vi "cloud_connection_arduino_uno.vi"() -> ()   [LabVIEW 2020]
uses:
  <vilib>/Skyline/Tag/Shared/typedefs/DataType.ctl
  <vilib>/Skyline/Tag/Wrapper/Wrapper_class/Tag Value Cluster Wrapper.ctl
  <vilib>/Skyline/Configuration/Configuration_class/NI Skyline Configuration.lvclass
  <vilib>/Skyline/Tag/Shared/typedefs/Tag Value Cluster.ctl
  <vilib>/Skyline/Tag/Wrapper/Wrapper_class/Generate Tag Cluster (DBL) 2.vi
  <vilib>/Skyline/Tag/Shared/Serialize Double to String.vi
  <vilib>/MakerHub/LINX/Public/Utilities/Open Serial.vi
  <vilib>/MakerHub/LINX/Public/Sensors/Motion/Servo/Servo Open One Channel.vi
  <vilib>/Skyline/Configuration/Configuration HTTP_class/Open Configuration API Key.vi
  <vilib>/Skyline/Tag/Wrapper/Wrapper_class/Configure Retention (Count).vi
  <vilib>/MakerHub/LINX/Public/Sensors/Motion/Servo/Servo Set Pulse Width One Channel.vi
  <vilib>/Utility/file.llb/Read Delimited Spreadsheet (DBL).vi
  <vilib>/Skyline/Tag/Wrapper/Wrapper_class/Generate Tag Cluster Core 2.vi
  <vilib>/MakerHub/LINX/Public/Sensors/Motion/Servo/Servo Close One Channel.vi
  <vilib>/Skyline/Tag/Wrapper/Wrapper_class/Close Tag (Multiple).vi
  <vilib>/Skyline/Configuration/Configuration HTTP_class/NI Skyline Configuration HTTP.lvclass
  <vilib>/Skyline/Tag/Wrapper/Wrapper HTTP_class/NI Skyline Tag HTTP.lvclass
  <vilib>/Skyline/Tag/Wrapper/Wrapper_class/NI Skyline Tag.lvclass
  <vilib>/Skyline/Tag/Shared/NI Skyline Tag.lvlib
  <vilib>/MakerHub/LINX/LMH-LINX.lvlib
  <vilib>/MakerHub/LINX/Public/Sensors/Motion/Servo/Servo.lvlib
panel:
  out "Angle1":dbl format="%#_3f"
  out "Angle2":dbl
  out "Angle 3":dbl
  in  "start 2":bool
  out "Error Out 2":errorcluster
  out "Error Out":errorcluster
  in  "Serial Port":refnum<visa-resource-name>="N/A"
  out "size(s)":i32
  out "subarray":dbl[](array[numeric])
  out "all rows":dbl[][](array[numeric])
  in  "start":bool
  in  "stop":bool
  in  "error in (no error)":errorcluster
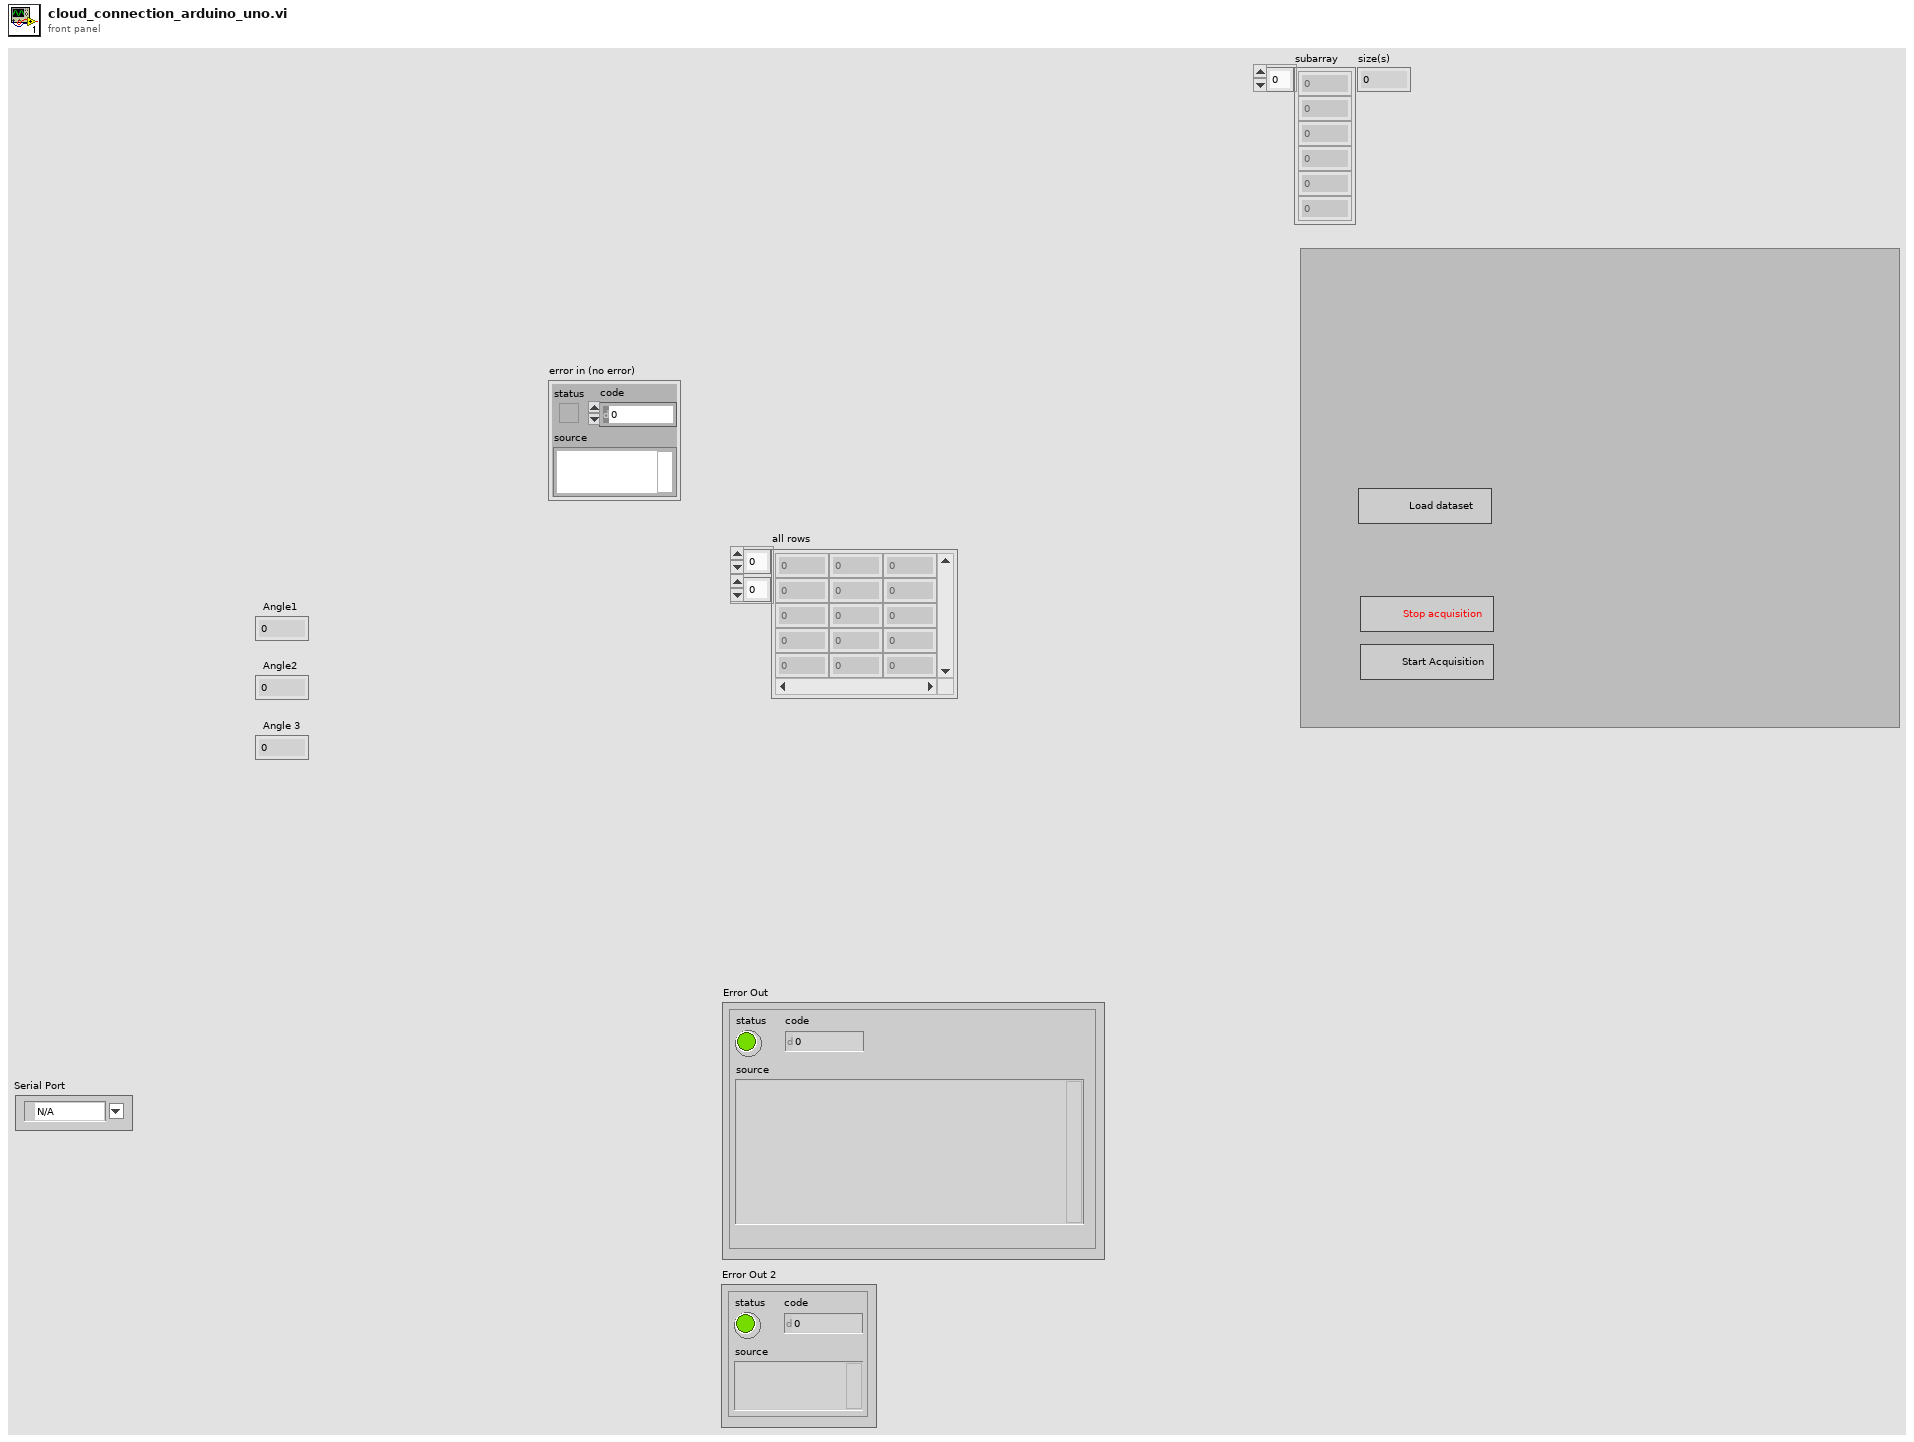
[diagram p1: front panel]
types:
  T1 = typedef "NI Skyline Tag.lvlib/DataType.ctl" = enum32{"Double", "I32", "String", "Boolean", "U64", "Timestamp"}
  T2 = typedef "LMH-LINX.lvlib/LINX Ref.ctl" = cluster{"IO":T3, "Interface":T4, "LINX Device Config":T5}
  T3 = typedef "LMH-LINX.lvlib/Platform.ctl" = enum16{"Remote", "Local"}
  T4 = typedef "LMH-LINX.lvlib/Interface.ctl" = enum16{"Serial", "TCP"}
  T5 = typedef "LMH-LINX.lvlib/Device.lvlib/LINX Device Config.ctl" = cluster{"Interface":T4, "COM Port":refnum<visa-resource-name>, "TCP Configuration":T6, "Device Family":u8, "Device ID":u8, "Device Name":string, "TCP Ref":refnum<k5>, "Channels":T7}
  T6 = typedef "LMH-LINX.lvlib/Device.lvlib/TCP Config.ctl" = cluster{"IP Address":string, "Port":u16}
  T7 = typedef "LMH-LINX.lvlib/Channels.ctl" = cluster{"DI":u8[], "DO":u8[], "AI":u8[], "AO":u8[], "PWM":u8[], "QE":u8[], "UART":u8[], "I2C 2":u8[], "SPI":u8[], "CAN":u8[], "Servo":u8[], "AI Ref (V)":dbl, "AI Resolution (Bits)":u8, "AO Ref (V)":dbl, "AO Resolution (Bits)":u8}
  T8 = typedef "NI Skyline Tag.lvclass/Tag Value Cluster Wrapper.ctl" = cluster{"Configuration":refnum<class "NI Skyline Configuration.lvclass">, "Tag Cluster":T9}
  T9 = typedef "NI Skyline Tag.lvlib/Tag Value Cluster.ctl" = cluster{"Path":string, "Workspace ID":string, "Data Type":T1, "Value":string, "Time Stamp":timestamp}
  T10 = cluster{"[0]":dbl, "[1]":dbl, "[2]":dbl, "[3]":dbl, "[4]":dbl, "[5]":dbl, "[6]":dbl, "[7]":dbl, "[8]":dbl}
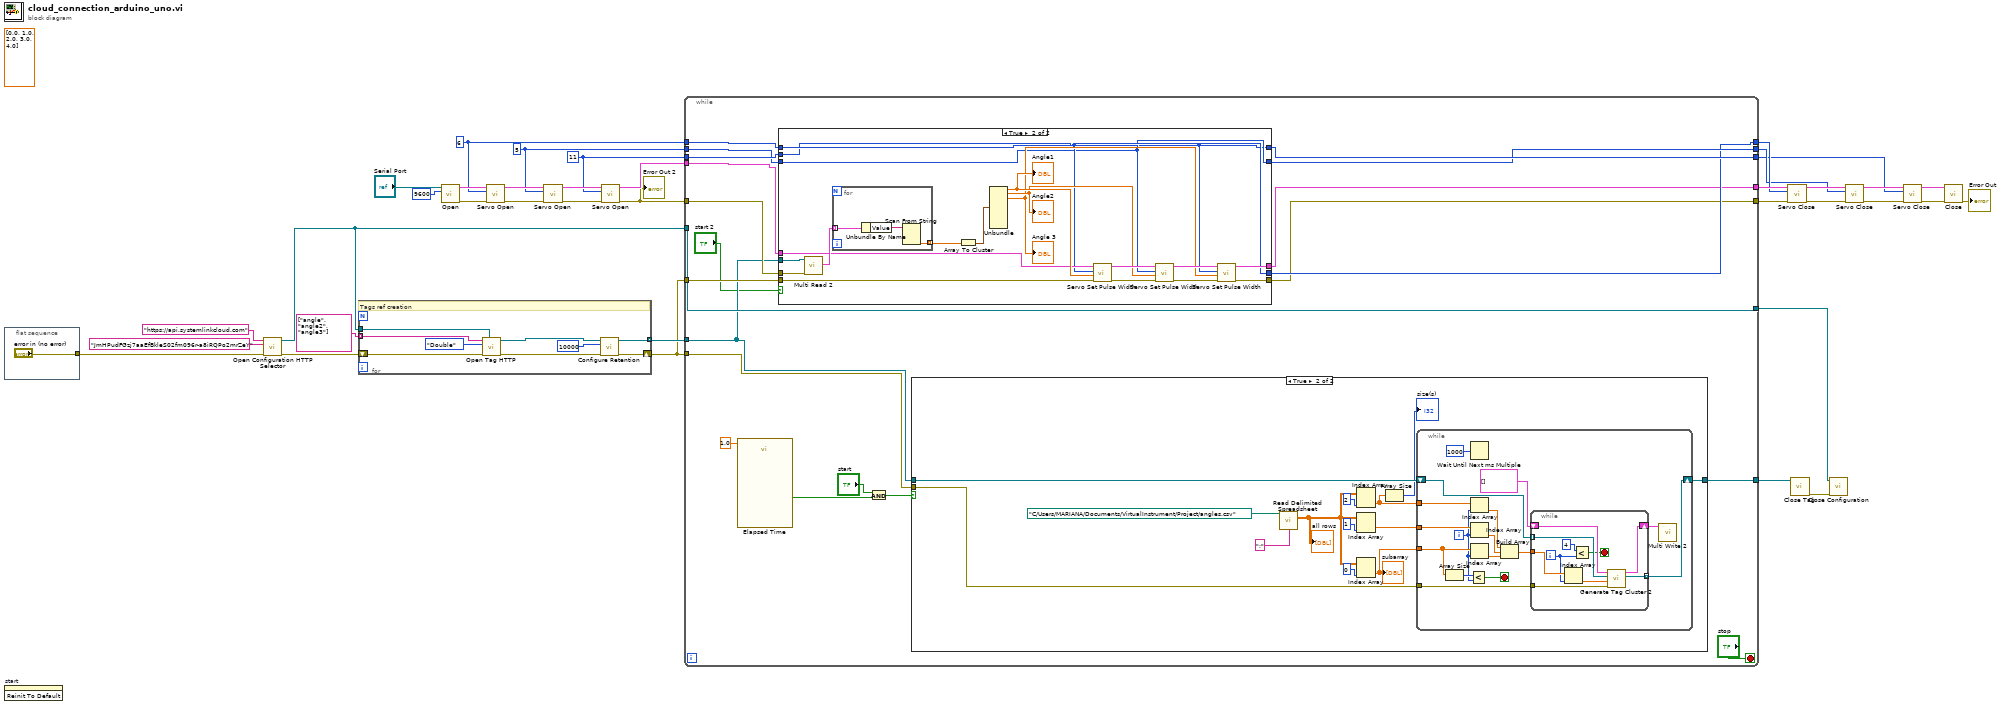
[diagram p0: block diagram]
diagram:
  w3 = u8 11 ("Servo Channel")
  w5 = u8 5 ("Servo Channel")
  w7 = u8 6 ("Servo Channel")
  (unwired) dbl[] [0.0, 1.0, 2.0, 3.0, 4.0]
  n1 = flat-sequence {
    tunnel: ["error in (no error)"] -> w34
    frame #0 {
    }
  }
  n2 = invoke on="start" class="Bool (strict)" method="Reinit To Default"() -> ()  [unwired: 3 in, 3 out]
  n3 = call-poly <vilib>:"Open Configuration HTTP Selector.vi"("error in (no error)"=w34, "api key"="JmHPudFGzj7aaEfBkleS02fm096r-a8iRQPo2mrZeY", "server url"="https://api.systemlinkcloud.com") -> ("error out"=w33:errorcluster, "configuration"=w30:refnum<class "NI Skyline Configuration HTTP.lvclass">)  [unwired: 7 in]
  n4 = for "Tags ref or creation" {
    tunnel: w30 -> [w46]
    tunnel: [w43] -> w29 mode=indexing
    tunnel: string[] ["angle", "angle2", "angle3"] -> [w38] mode=indexing
    shift-right: [w39] -> w1
    shift-left: w33 -> [w42]
    # "Tags ref creation"
    n5 = call <vilib>:"Open Tag HTTP.vi"("configuration"=w46, "error in (no error)"=w42, "Data Type"=DataType."Double", "path"=w38) -> ("error out"=w40:errorcluster, "tag"=w45:refnum<class "NI Skyline Tag.lvclass">)  [unwired: 6 in]
    n6 = call-poly <vilib>:"Configure Retention.vi"("error in (no error)"=w40, "maximum count"=u32 10000, "tag in"=w45) -> ("error out"=w39:errorcluster, "tag out"=w43:refnum<class "NI Skyline Tag.lvclass">)  [unwired: 7 in]
  }
  n7 = call-poly <vilib>:"Open.vi"("Baud Rate Override"=u32 9600, "Serial Port"="Serial Port") -> ("Error Out"=w25:errorcluster, "LINX Resource"=w26:T2)  [unwired: 7 in, 1 out]
  n8 = call-poly <vilib>:"Servo Open.vi"("Error In"=w25, "Servo Channel"=w7, "LINX Resource"=w26) -> ("Error Out"=w21:errorcluster, "LINX Resource"=w22:T2)  [unwired: 7 in]
  n9 = call-poly <vilib>:"Servo Open.vi"("Error In"=w21, "Servo Channel"=w5, "LINX Resource"=w22) -> ("Error Out"=w16:errorcluster, "LINX Resource"=w17:T2)  [unwired: 7 in]
  n10 = call-poly <vilib>:"Servo Open.vi"("Error In"=w16, "Servo Channel"=w3, "LINX Resource"=w17) -> ("Error Out"=w8:errorcluster, "LINX Resource"=w9:T2)  [unwired: 7 in]
  "Error Out 2" <- w8
  n11 = while {
    tunnel: [w67] -> w31
    tunnel: w30 -> [w67]
    tunnel: w1 -> [w60]
    tunnel: w29 -> [w53]
    tunnel: [w66] -> w27
    tunnel: [w49] -> w11
    tunnel: [w48] -> w10
    tunnel: w9 -> [w56]
    tunnel: w8 -> [w55]
    tunnel: w7 -> [w57]
    tunnel: [w50] -> w6
    tunnel: w5 -> [w58]
    tunnel: [w51] -> w4
    tunnel: w3 -> [w59]
    tunnel: [w52] -> w2
    tunnel: w1 -> [w54]
    stop <- "stop" stop-if-true
    n12 = call "Elapsed Time"("Time Target (s)"=1.0) -> ("Time has Elapsed"=w62:bool)  [unwired: 11 in, 7 out]
    n13 = case shown="True" "start 2" {
      tunnel: w53 -> [_ w89]
      tunnel: w55 -> [_ w87]
      tunnel: w59 -> [w70 w73]
      tunnel: w58 -> [w69 w74]
      tunnel: w57 -> [w68 w75]
      tunnel: w56 -> [w72 w79]
      tunnel: w54 -> [w71 w78]
      tunnel: [w72 w77] -> w49
      tunnel: [w71 w76] -> w48
      tunnel: [w70 w75] -> w50
      tunnel: [w69 w74] -> w51
      tunnel: [w68 w73] -> w52
      frame False {
      }
      frame True {
        n14 = call <vilib>:"Multi Read 2.vi"("error in (no error)"=w87, "tags in"=w89) -> ("tag clusters"=w88:T9[])  [unwired: 7 in, 2 out]
        n15 = for {
          tunnel: [w94] -> w91 mode=indexing
          tunnel: w88 -> [w92] mode=indexing
          n16 = Unbundle By Name(w92) -> ("Value"=w93:string)
          n17 = Scan From String(input string=w93) -> (output 1=w94:dbl)  [unwired: 4 in, 3 out]
        }
        n18 = Array To Cluster(array=w91) -> (cluster=w90:T10)
        n19 = Unbundle(w90) -> ("[0]"=w82:dbl, "[1]"=w81:dbl, "[2]"=w80:dbl)  [unwired: 6 out]
        "Angle1" <- w82
        "Angle2" <- w81
        "Angle 3" <- w80
        n20 = call-poly <vilib>:"Servo Set Pulse Width.vi"("Error In"=w78, "Pulse Width (uS)"=w82, "Servo Channel"=w75, "LINX Resource"=w79) -> ("Error Out"=w85:errorcluster, "LINX Resource"=w86:T2)  [unwired: 6 in]
        n21 = call-poly <vilib>:"Servo Set Pulse Width.vi"("Error In"=w85, "Pulse Width (uS)"=w81, "Servo Channel"=w74, "LINX Resource"=w86) -> ("Error Out"=w83:errorcluster, "LINX Resource"=w84:T2)  [unwired: 6 in]
        n22 = call-poly <vilib>:"Servo Set Pulse Width.vi"("Error In"=w83, "Pulse Width (uS)"=w80, "Servo Channel"=w73, "LINX Resource"=w84) -> ("Error Out"=w76:errorcluster, "LINX Resource"=w77:T2)  [unwired: 6 in]
      }
    }
    n23 = And(x="start", y=w62) -> (x .and. y?=w61:bool)
    n24 = case shown="True" w61 {
      tunnel: w60 -> [_ w107]
      tunnel: w53 -> [w95 w106]
      tunnel: [w95 w108] -> w66
      frame False {
      }
      frame True {
        n25 = call-poly <vilib>:"Read Delimited Spreadsheet.vi"("file path (dialog if empty)"=path "C:/Users/MARIANA/Documents/VirtualInstrument/Project/angles.csv", "delimiter (\\t)"=";" ("delimiter (\\t)")) -> ("all rows"=w101:dbl[][])  [unwired: 8 in, 5 out]
        "all rows" <- w101
        n26 = Index Array(array=w101, index (col)=2 ("index")) -> (element=w97:dbl[])  [unwired: 1 in]
        n27 = Index Array(array=w101, index (col)=1 ("index")) -> (element=w100:dbl[])  [unwired: 1 in]
        n28 = Index Array(array=w101, index (col)=0 ("disabled index (col)")) -> (element=w102:dbl[])  [unwired: 1 in]
        "subarray" <- w102
        n29 = Array Size(array=w97) -> (size(s)=→"size(s)":i32)
        n30 = while {
          tunnel: w107 -> [w122]
          shift-right: [w123] -> w108
          shift-left: w106 -> [w120]
          tunnel: w102 -> [w116]
          tunnel: w100 -> [w112]
          tunnel: w97 -> [w111]
          i -> [w109]
          stop <- w118 stop-if-true
          n31 = Array Size(array=w116) -> (size(s)=w117:i32)
          n32 = Less?(x=w117, y=w109) -> (x < y?=w118:bool)
          n33 = Wait Until Next ms Multiple(millisecond multiple=u32 1000) -> ()  [unwired: 1 out]
          n34 = Index Array(array=w111, index=w109) -> (element=w110:dbl)
          n35 = Index Array(array=w112, index=w109) -> (element=w113:dbl)
          n36 = Index Array(array=w116, index=w109) -> (element=w114:dbl)
          n37 = Build Array(w110, w113, w114) -> (w119:dbl[])
          n38 = while {
            shift-right: [w134] -> w124
            shift-left: T8[] [] ("tag clusters in") -> [w131]
            tunnel: [w133] -> w123 mode=indexing
            tunnel: w122 -> [w132]
            tunnel: w120 -> [w130] mode=indexing
            tunnel: w119 -> [w128]
            i -> [w127]
            stop <- w125 stop-if-true
            n39 = Index Array(array=w128, index=w127) -> (element=w129:dbl)
            n40 = Less?(x=4, y=w127) -> (x < y?=w125:bool)
            n41 = call-poly <vilib>:"Generate Tag Cluster 2.vi"("error in (no error)"=w132, "value"=w129, "tag in"=w130, "tag clusters in"=w131) -> ("tag out"=w133:refnum<class "NI Skyline Tag.lvclass">, "tag clusters out"=w134:T8[])  [unwired: 5 in, 1 out]
          }
          n42 = call <vilib>:"Multi Write 2.vi"("tag clusters"=w124) -> ()  [unwired: 10 in, 1 out]
        }
      }
    }
  }
  n43 = call-poly <vilib>:"Servo Close.vi"("Error In"=w10, "Servo Channel"=w6, "LINX Resource"=w11) -> ("Error Out"=w19:errorcluster, "LINX Resource"=w20:T2)  [unwired: 7 in]
  n44 = call-poly <vilib>:"Close Tag.vi"("tags"=w27) -> ("error out"=w32:errorcluster)  [unwired: 10 in]
  n45 = call-dynamic "Close Configuration.vi"("error in (no error)"=w32, "configuration"=w31) -> ()  [unwired: 9 in, 1 out]
  n46 = call-poly <vilib>:"Servo Close.vi"("Error In"=w19, "Servo Channel"=w4, "LINX Resource"=w20) -> ("Error Out"=w14:errorcluster, "LINX Resource"=w15:T2)  [unwired: 7 in]
  n47 = call-poly <vilib>:"Servo Close.vi"("Error In"=w14, "Servo Channel"=w2, "LINX Resource"=w15) -> ("Error Out"=w12:errorcluster, "LINX Resource"=w13:T2)  [unwired: 7 in]
  n48 = call <vilib>:"Close.vi"("Error In"=w12, "LINX Resource"=w13) -> ("Error Out"=→"Error Out":errorcluster)  [unwired: 9 in]
